vi "Write Next Tag.vi"(8 "error in (no error)":errorcluster, 10 "Next Tag":u64, 11 "Tree Manager in":refnum<class "Tree Manager.lvclass">) -> (0 "error out":errorcluster, 3 "Tree Manager out":refnum<class "Tree Manager.lvclass">)   [LabVIEW 2026, in "VILab.lvlib" / "Tree Manager.lvclass"]
uses:
  Tree Manager.lvclass
  Tree Manager.lvclass/Tree Manager.ctl
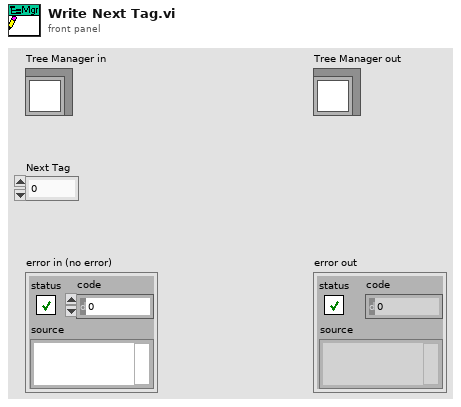
[diagram p1: front panel]
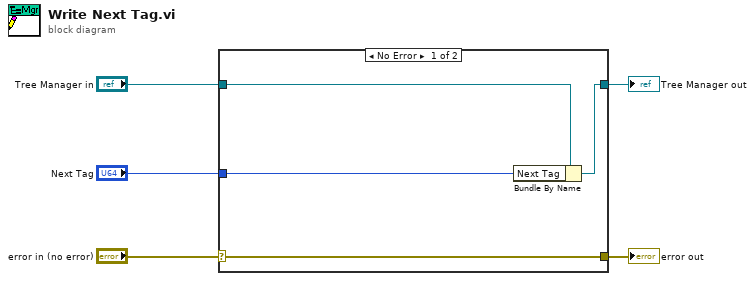
[diagram p0: block diagram]
diagram:
  n1 = case shown="No Error" "error in (no error)" {
    selector: "error in (no error)" -> [w9 w10]
    tunnel: [w9 w10] -> w4
    tunnel: [w7 w11] -> w2
    tunnel: "Tree Manager in" -> [w8 w11]
    tunnel: "Next Tag" -> [w6 _]
    frame No Error {
      n2 = Bundle By Name(cluster=w8, "Next Tag"=w6) -> (w7:refnum<class "Tree Manager.lvclass">)
    }
    frame Error {
    }
  }
  "error out" <- w4
  "Tree Manager out" <- w2
